vi "Format Message Log Data.vi"(11 "Message Data":T1) -> (3 "Array":string[](array[string]))   [LabVIEW 2017, in "Message Log.lvclass"]
uses:
  Message Log.lvclass
  <vilib>/addons/_Workers/Library/Classes/Worker/Debug Message Data.ctl
  <vilib>/addons/_Workers/Library/Classes/Message/Message Time Stamp.ctl
  <vilib>/addons/_Workers/Library/Case Label.ctl
  <vilib>/addons/_Workers/Library/Classes/Message/Priority (ALL).ctl
  <vilib>/addons/_Workers/Library/Classes/Message/Message.lvclass
  <vilib>/addons/_Workers/Library/Workers.lvlib
  <vilib>/addons/_Workers/Library/Classes/Worker/Worker.lvclass
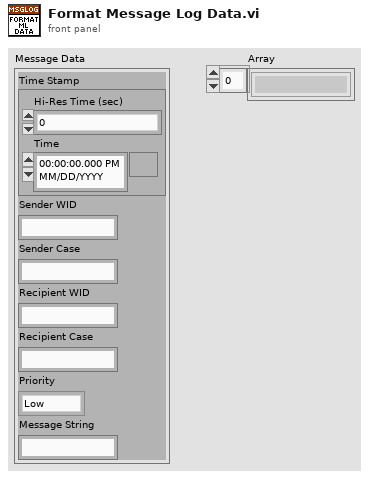
[diagram p1: front panel]
types:
  T1 = typedef "Workers.lvlib/Worker.lvclass/Debug Message Data.ctl" = cluster{"Time Stamp":T2, "Sender WID":string, "Sender Case":T3, "Recipient WID":string, "Recipient Case":T3, "Priority":T4, "Message String":string}
  T2 = typedef "Workers.lvlib/Message.lvclass/Message Time Stamp.ctl" = cluster{"Hi-Res Time (sec)":dbl, "Time":timestamp}
  T3 = typedef "Workers.lvlib/Case Label.ctl" = string
  T4 = typedef "Workers.lvlib/Message.lvclass/Priority (ALL).ctl" = enum16{"Low", "Normal", "High", "Critical"}
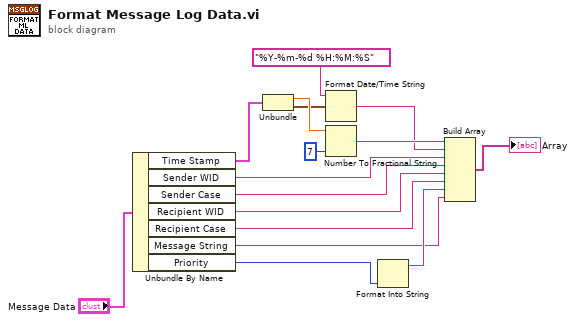
[diagram p0: block diagram]
diagram:
  n1 = Unbundle By Name("Message Data") -> ("Time Stamp"=w9:T2, "Sender WID"=w6:string, "Sender Case"=w5:T3, "Recipient WID"=w4:string, "Recipient Case"=w2:T3, "Message String"=w3:string, "Priority"=w13:T4)
  n2 = Unbundle(w9) -> ("Hi-Res Time (sec)"=w12:dbl, "Time"=w11:timestamp)
  n3 = Format Date/Time String(time format string (%c)="%Y-%m-%d %H:%M:%S", seconds (now)=w11) -> (date/time string=w7:string)  [unwired: 1 out]
  n4 = Number To Fractional String(number=w12, precision (6)=i16 7) -> (F-format string=w8:string)  [unwired: 2 in]
  n5 = Format Into String(w13) -> (resulting string=w14:string)  [unwired: 3 in, 1 out]
  n6 = Build Array(w8, w7, w6, w5, w4, w2, w14, w3) -> (→"Array":T3[])
